vi "EventStart.vi"(7 "Event Name":string, 8 "error in":errorcluster) -> (0 "error out":errorcluster)   [LabVIEW 2026, in "VS_Perfetto.lvlib"]
uses:
  VS_Perfetto.lvlib
  libvs_perfetto.dll
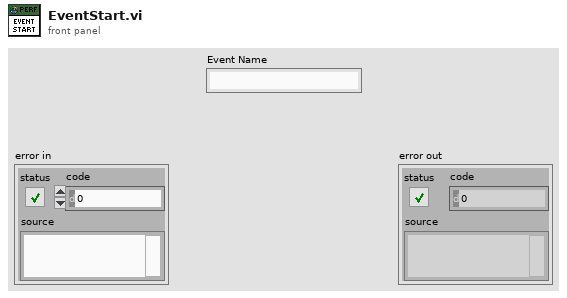
[diagram p1: front panel]
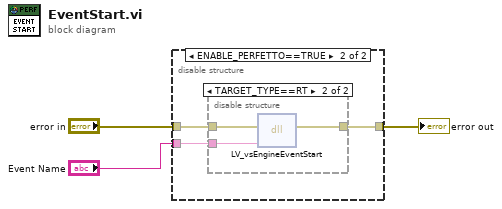
[diagram p0: block diagram]
diagram:
  n1 = disable-structure shown="ENABLE_PERFETTO==TRUE" {
    disable-tunnel: "Event Name" -> [_ w5]
    disable-tunnel: "error in" -> [w4 w6]
    disable-tunnel: [w4 w7] -> w2
    frame condition #0 (active) {
    }
    frame condition #1 {
      n2 = disable-structure shown="TARGET_TYPE==RT" {
        disable-tunnel: [w8 w11] -> w7
        disable-tunnel: w6 -> [w8 w10]
        disable-tunnel: w5 -> [_ w9]
        frame condition #0 (active) {
        }
        frame condition #1 {
          n3 = dll-call lib="libvs_perfetto.*" fn="LV_vsEngineEventStart"(error in=w10, "eventName"=w9) -> (error out=w11:errorcluster)  [unwired: 4 in, 1 out]
        }
      }
    }
  }
  "error out" <- w2
